vi "Defragment All tdms in a folder.vi"() -> ()   [LabVIEW 2020]
uses:
  <vilib>/regexp/Match Regular Expression.xnode
panel:
  out "String":string
  out "filenames":string[](array[string])
  out "Tdms list":path[](array[path])
  out "error out":errorcluster
  out "Check":string[](array[string])
  in  "Folder Path":path
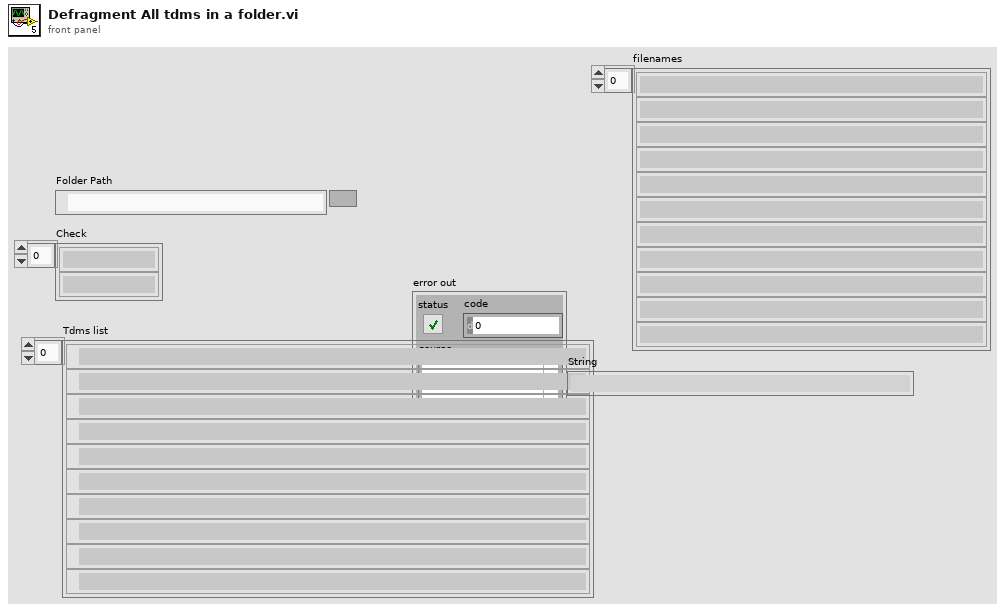
[diagram p1: front panel]
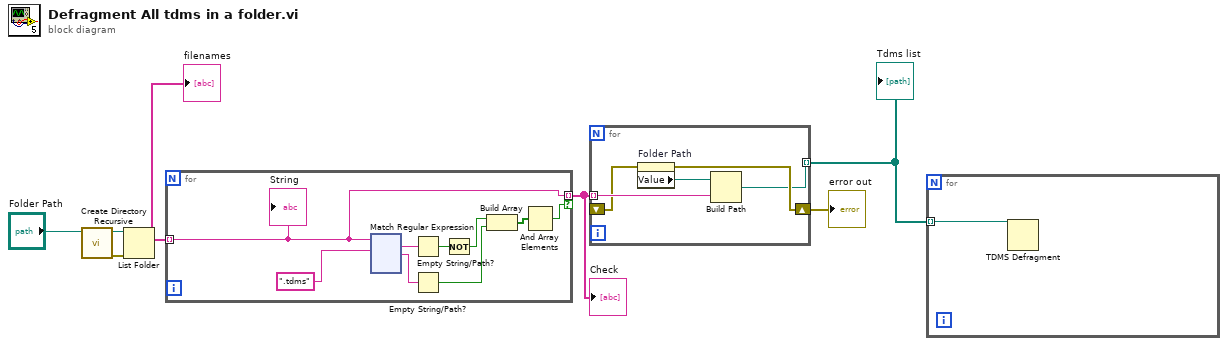
[diagram p0: block diagram]
diagram:
  n1 = call <vilib>:"Create Directory Recursive.vi"("directory"="Folder Path") -> ("error out"=w4:errorcluster, "directory copy"=w6:path)  [unwired: 4 in, 1 out]
  n2 = List Folder(path=w6, error in=w4) -> (filenames=w5:string[])  [unwired: 2 in, 3 out]
  "filenames" <- w5
  n3 = for {
    tunnel: w5 -> [w8] mode=indexing
    tunnel: [w8] -> w3 mode=indexing if=w10
    n4 = xnode "Match Regular Expression"("input string"=w8, "regular expression"=".tdms") -> ("whole match"=w11:string, "after match"=w16:string)  [unwired: 4 in, 3 out]
    n5 = Empty String/Path?(string/path=w11) -> (empty?=w15:bool)
    n6 = Empty String/Path?(string/path=w16) -> (empty?=w13:bool)
    n7 = Not(x=w15) -> (.not. x?=w14:bool)
    n8 = Build Array(w14, w13) -> (w12:bool[])
    n9 = And Array Elements(Boolean array=w12) -> (logical AND=w10:bool)
    "String" <- w8
  }
  "Check" <- w3
  n10 = for {
    tunnel: w3 -> [w134] mode=indexing
    shift-right: [w132] -> w2
    shift-left: _ -> [w133]
    tunnel: [w131] -> w1 mode=indexing
    n11 = property on="Folder Path" class="Path"(error in=w133) -> (error out=w132:errorcluster, "Value"=w135:path)  [unwired: 1 in, 1 out]
    n12 = Build Path(base path=w135, name or relative path=w134) -> (appended path=w131:path)
  }
  "error out" <- w2
  "Tdms list" <- w1
  n13 = for {
    tunnel: w1 -> [w136] mode=indexing
    n14 = TDMS Defragment(7:w136) -> ()  [unwired: 1 in, 1 out]
  }
